vi "Read Node Type.vi"(8 "error in (no error)":errorcluster, 11 "Picture Ring in":refnum<class "Picture Ring.lvclass">) -> (0 "error out":errorcluster, 2 "Node Type":T1, 3 "Picture Ring out":refnum<class "Picture Ring.lvclass">)   [LabVIEW 2019, in "Picture Ring.lvclass"]
uses:
  Picture Ring.lvclass
  Node Type--enum.ctl
  Picture Ring.lvclass/Picture Ring.ctl
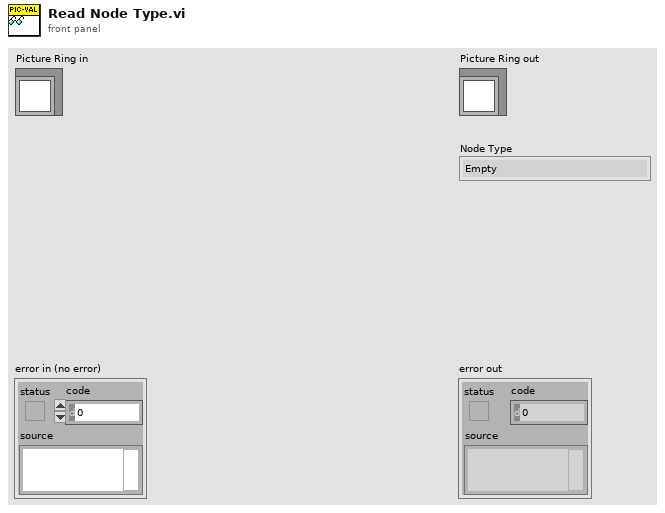
[diagram p1: front panel]
types:
  T1 = typedef "Picture Ring.lvclass/Node Type--enum.ctl" = enum16{"Empty", "Blocked", "Start", "End", "Path"}
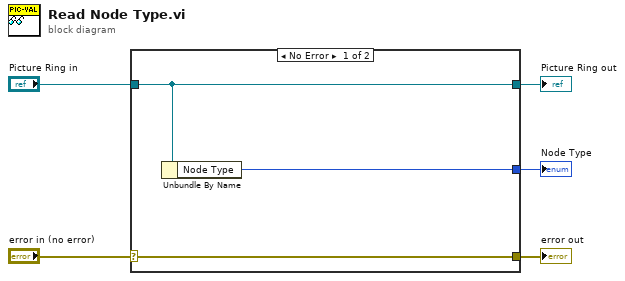
[diagram p0: block diagram]
diagram:
  n1 = case shown="No Error" "error in (no error)" {
    selector: "error in (no error)" -> [w8 w9]
    tunnel: [w8 w9] -> w4
    tunnel: [w7 w10] -> w2
    tunnel: "Picture Ring in" -> [w7 w10]
    tunnel: [w6 _] -> w1
    frame No Error {
      n2 = Unbundle By Name(w7) -> ("Node Type"=w6:T1)
    }
    frame Error {
    }
  }
  "error out" <- w4
  "Picture Ring out" <- w2
  "Node Type" <- w1
